vi "公约数.vi"(10 "数值 2":dbl, 11 "数值":dbl) -> (2 "下拉列表":u16(ring) items=["1", "5"], 3 "数组":i32[](array[numeric]))   [LabVIEW 2019]
panel:
  out "x+1":i32
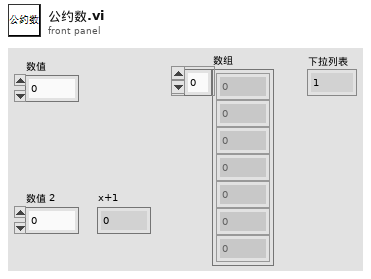
[diagram p1: front panel]
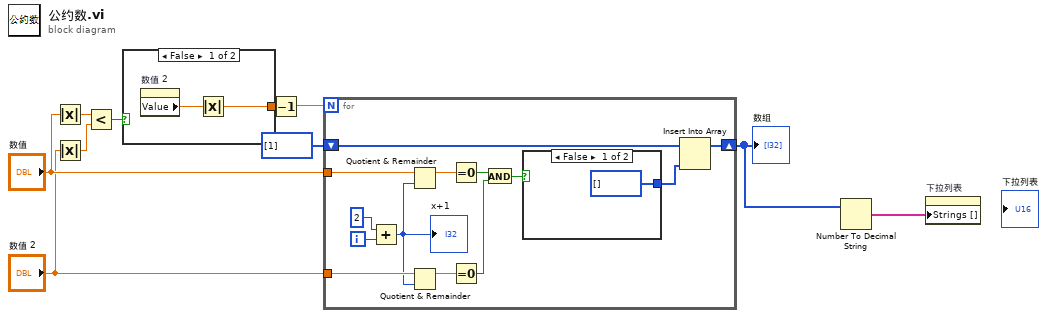
[diagram p0: block diagram]
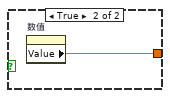
[diagram p2: hidden frame]
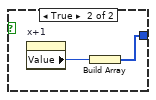
[diagram p3: hidden frame]
diagram:
  n1 = Absolute Value(x="数值") -> (abs(x)=w8:dbl)
  n2 = Absolute Value(x="数值 2") -> (abs(x)=w7:dbl)
  n3 = Less?(x=w8, y=w7) -> (x < y?=w10:bool)
  n4 = case shown="False" w10 {
    tunnel: [w11 w13] -> w9
    frame False {
      n5 = property on="数值 2" class="DigNum (strict)"() -> ("Value"=w12:dbl)  [unwired: 2 in, 2 out]
      n6 = Absolute Value(x=w12) -> (abs(x)=w11:dbl)
    }
    frame True {
      n7 = property on="数值" class="DigNum (strict)"() -> ("Value"=w13:dbl)  [unwired: 2 in, 2 out]
    }
  }
  n8 = Decrement(x=w9) -> (x-1=w4:dbl)
  n9 = for {
    N: w4 -> [_]
    tunnel: "数值" -> [w25]
    tunnel: "数值 2" -> [w24]
    shift-right: [w15] -> w2
    shift-left: i32[] [1] ("数组") -> [w16]
    i -> [w26]
    n10 = Add(x=2, y=w26) -> (x+y=w18:i32)
    "x+1" <- w18
    n11 = Quotient & Remainder(x=w25, y=w18) -> (x-y*floor(x/y)=w23:dbl)  [unwired: 1 out]
    n12 = Quotient & Remainder(x=w24, y=w18) -> (x-y*floor(x/y)=w22:dbl)  [unwired: 1 out]
    n13 = Equal To 0?(x=w23) -> (x = 0?=w21:bool)
    n14 = Equal To 0?(x=w22) -> (x = 0?=w20:bool)
    n15 = And(x=w21, y=w20) -> (x .and. y?=w19:bool)
    n16 = case shown="False" w19 {
      tunnel: [i32[] [] w28] -> w14
      frame False {
      }
      frame True {
        n17 = property on="x+1" class="DigNum (strict)"() -> ("Value"=w29:i32)  [unwired: 2 in, 2 out]
        n18 = Build Array(w29) -> (w28:i32[])
      }
    }
    n19 = Insert Into Array(array=w16, new element=w14) -> (w15:i32[])  [unwired: 1 in]
  }
  "数组" <- w2
  n20 = Number To Decimal String(number=w2) -> (decimal integer string=w1:string[])  [unwired: 1 in]
  n21 = property on="下拉列表" class="Ring (strict)"("Strings []"=w1) -> ()  [unwired: 2 in, 2 out]
